vi "H5Gget_linkval.vi"(6 "error in (no error)":errorcluster, 8 "Name":string, 9 "HDF5 Ref":T1) -> (0 "error out":errorcluster, 2 "Value":string, 3 "HDF5 Ref out":T1)   [LabVIEW 2017]
doc: "Returns the name of the object that the symbolic link points to."
uses:
  <vilib>/UPVI/lvhdf5/library.llb/HDF5 Ref.ctl
  <vilib>/UPVI/lvhdf5/hdf5.dll
panel:
  # "LVHDF5 Toolkit\nCopyright (c) 2005-2013 by Jason D. Sommerville\nCopyright (c) 2014 by UPVI, LLC.\n\nThis use and distribution of this file is governed by the terms found in \nLICENSE.txt distributed with this toolkit and installed at\n <user.lib>\\_lvhdf5\\LICENSE.txt"
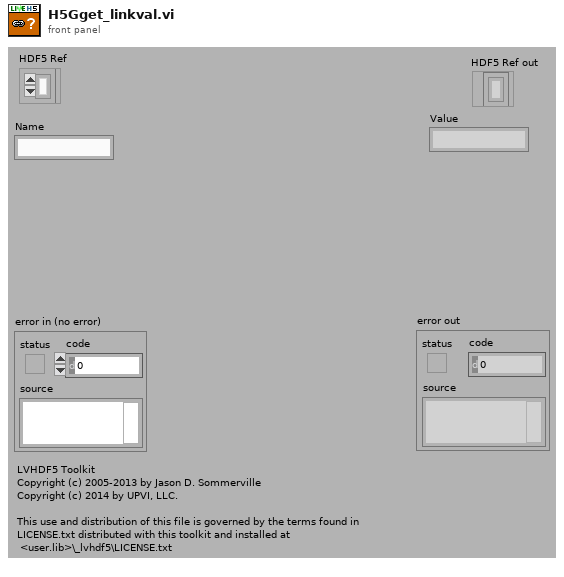
[diagram p1: front panel]
types:
  T1 = typedef "HDF5 Ref.ctl" = refnum<k1>
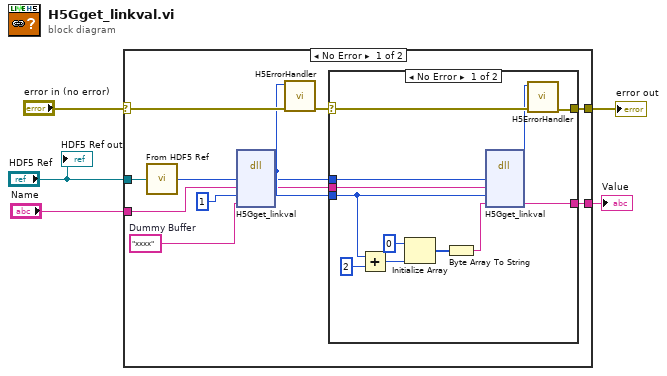
[diagram p0: block diagram]
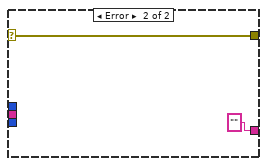
[diagram p2: hidden frame]
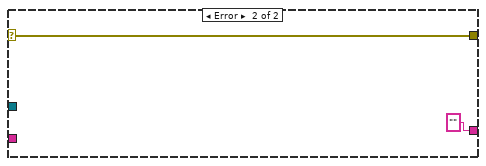
[diagram p3: hidden frame]
diagram:
  n1 = case shown="No Error" "error in (no error)" {
    selector: "error in (no error)" -> [w17 w33]
    tunnel: [w13 w33] -> w4
    tunnel: "HDF5 Ref" -> [w16 _]
    tunnel: "Name" -> [w8 _]
    tunnel: [w9 "" ("name")] -> w1
    frame No Error {
      w7 = "xxxx"  # Dummy Buffer
      n2 = call <vilib>:"From HDF5 Ref.vi"("HDF5 Ref"=w16) -> ("I32"=w15:i32)
      n3 = dll-call lib="C:/Program Files/National Instruments/LabVIEW 2017/vi.lib/UPVI/lvhdf5/hdf5.dll" fn="H5Gget_linkval"("loc_id"=w15, "name"=w8, "size"=u32 1, "value"=w7) -> ("return type"=w12:i32, "loc_id"=w10:i32, "name"=w11:string)  [unwired: 5 in, 2 out]
      n4 = call <vilib>:"H5ErrorHandler.vi"("error in (no error)"=w17, "herr_t"=w12) -> ("error out"=w14:errorcluster)  [unwired: 3 in, 4 out]
      n5 = case shown="No Error" w14 {
        selector: w14 -> [w24 w31]
        tunnel: [w25 w31] -> w13
        tunnel: w12 -> [w22 _]
        tunnel: w11 -> [w21 _]
        tunnel: w10 -> [w20 _]
        tunnel: [w18 "" ("name")] -> w9
        frame No Error {
          n6 = Add(x=w22, y=2) -> (x+y=w27:i32)
          n7 = Initialize Array(u8 0, w27) -> (w26:u8[])
          n8 = Byte Array To String(unsigned byte array=w26) -> (string=w23:string)
          n9 = dll-call lib="C:/Program Files/National Instruments/LabVIEW 2017/vi.lib/UPVI/lvhdf5/hdf5.dll" fn="H5Gget_linkval"("loc_id"=w20, "name"=w21, "size"=w22, "value"=w23) -> ("return type"=w19:i32, "value"=w18:string)  [unwired: 6 in, 2 out]
          n10 = call <vilib>:"H5ErrorHandler.vi"("error in (no error)"=w24, "herr_t"=w19) -> ("error out"=w25:errorcluster)  [unwired: 3 in, 4 out]
        }
        frame Error {
        }
      }
    }
    frame Error {
    }
  }
  "error out" <- w4
  "Value" <- w1
  "HDF5 Ref out" <- "HDF5 Ref"
